vi "Relay.vi"(8 "error in":errorcluster, 10 "Test":T1, 11 "DIO ID":string) -> (0 "error out":errorcluster={"status"=TRUE, "code"=1446, "source"="Preserve Run-Time Class in MAL.lvlib:Relay.vi"})   [LabVIEW 2025, in "Submodule EOL.lvlib" / "Submodule EOL.lvclass"]
uses:
  Submodule EOL.lvclass
  Test.ctl
  Users/Public/Documents/Sandia National Labs/TSS Plugin/Engines/Digital IO.lvlibp/Digital IO Instrument/Digital IO Instrument.lvclass
  Submodule EOL.lvclass/Submodule EOL.ctl
  Users/Public/Documents/Sandia National Labs/TSS Plugin/CEF.lvlibp/Node/CEF_Node.lvclass
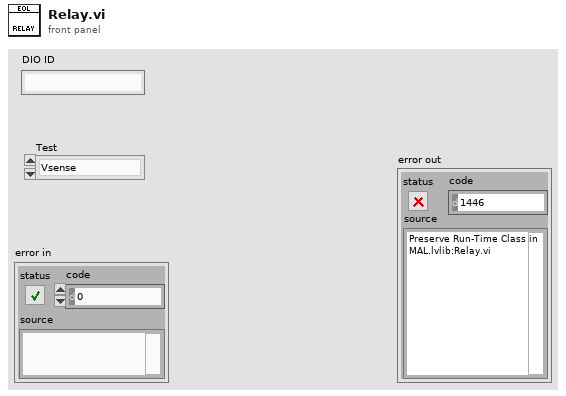
[diagram p1: front panel]
types:
  T1 = typedef "Submodule EOL.lvlib/Submodule EOL.lvclass/Test.ctl" = enum16{"Vsense", "Thermistor", "ACIR", "HiPOT1", "HiPOT2"}
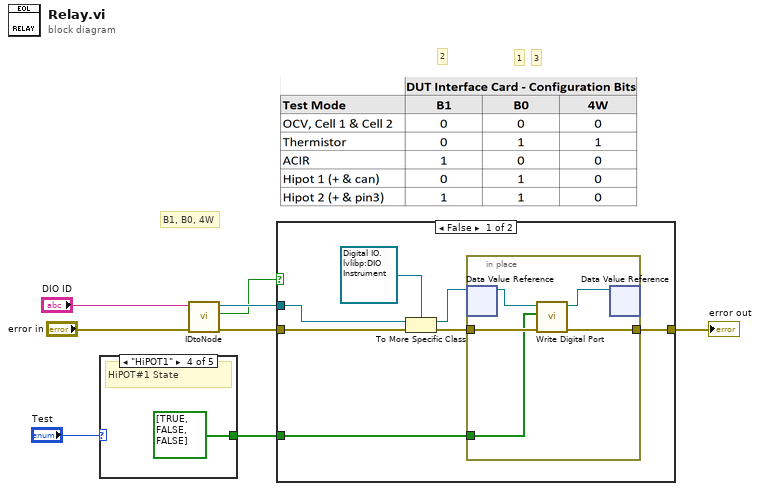
[diagram p0: block diagram]
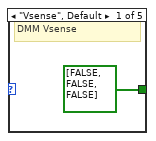
[diagram p2: hidden frame]
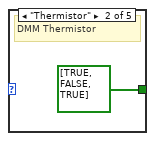
[diagram p3: hidden frame]
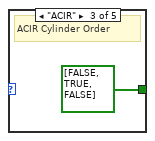
[diagram p4: hidden frame]
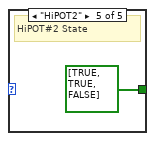
[diagram p5: hidden frame]
diagram:
  # "3"
  # "2"
  # "1"
  # "B1, B0, 4W"
  n1 = case shown="\"HiPOT1\"" "Test" {
    tunnel: [bool[] [FALSE, FALSE, FALSE] bool[] [TRUE, FALSE, TRUE] bool[] [FALSE, TRUE, FALSE] bool[] [TRUE, FALSE, FALSE] bool[] [TRUE, TRUE, FALSE]] -> w1
    frame "Vsense", Default {
      # "DMM Vsense"
    }
    frame "Thermistor" {
      # "DMM Thermistor"
    }
    frame "ACIR" {
      # "ACIR Cylinder Order"
    }
    frame "HiPOT1" {
      # "HiPOT#1 State"
    }
    frame "HiPOT2" {
      # "HiPOT#2 State"
    }
  }
  n2 = call "IDtoNode.vi"("error in"="error in", "ID"="DIO ID") -> ("error out"=w7:errorcluster, "invalid Id"=w4:bool, "node ref"=w6:refnum<data-value>)  [unwired: 7 in]
  n3 = case shown="False" w4 {
    tunnel: w7 -> [w20 w26]
    tunnel: w6 -> [w19 _]
    tunnel: w1 -> [w14 _]
    tunnel: [w15 w26] -> w3
    frame False {
      n4 = To More Specific Class(target class=refnum<data-value> refnum, reference=w19, error in=w20) -> (specific class reference=w17:refnum<data-value>, error out=w16:errorcluster)
      n5 = in-place {
        in-place-border: w16 -> [w25]
        in-place-border: [w23] -> w15
        in-place-border: w14 -> [w22]
        n6 = in-place-dvr #1(w17) -> (w24:refnum<class "Digital IO Instrument.lvclass">)  [unwired: 1 out]
        n7 = call-dynamic "Write Digital Port.vi"("error in (no error)"=w25, "DOs"=w22, "Digital Output in"=w24) -> ("error out"=w23:errorcluster, "Digital Output out"=w21:refnum<class "Digital IO Instrument.lvclass">)  [unwired: 7 in]
        n8 = in-place-dvr #1(w21) -> ()  [unwired: 2 out]
      }
    }
    frame True {
    }
  }
  "error out" <- w3
